vi "Retrieve Stored Session.vi"(8 "error in (no error)":errorcluster, 10 "Session in":refnum<class "Session.lvclass">, 11 "Client ID":string) -> (0 "error out":errorcluster, 1 "found":bool, 2 "Retrieved Session":refnum<class "Session.lvclass">)   [LabVIEW 2013, in "MQTT Server.lvlib" / "StoredSessions.lvclass"]
uses:
  StoredSessions.lvclass
  <vilib>/LabVIEW Open Source Project/MQTT Connection/MQTT_Base/Session/Session.lvclass
  <vilib>/LabVIEW Open Source Project/MQTT Connection/MQTT_Base/Session/Session State -- cluster.ctl
  <vilib>/LabVIEW Open Source Project/MQTT Control Packets/Control Packets/SUBSCRIBE/Topic Subscription -- cluster.ctl
  <vilib>/LabVIEW Open Source Project/MQTT Control Packets/Control Packets/ControlPacket/QualityOfService -- enum.ctl
  <vilib>/LabVIEW Open Source Project/MQTT Control Packets/Control Packets/ControlPacket/Pending Transmission -- cluster.ctl
  <vilib>/LabVIEW Open Source Project/MQTT Control Packets/Control Packets/ControlPacket/ControlPacket.lvclass
  <vilib>/LabVIEW Open Source Project/MQTT Connection/MQTT_Base/Session/Pending ACKs -- cluster.ctl
  <vilib>/LabVIEW Open Source Project/MQTT Connection/MQTT_Base/Session/Session.lvclass/Session.ctl
  <vilib>/LabVIEW Open Source Project/MQTT Control Packets/Control Packets/SUBSCRIBE/SUBSCRIBE.lvclass
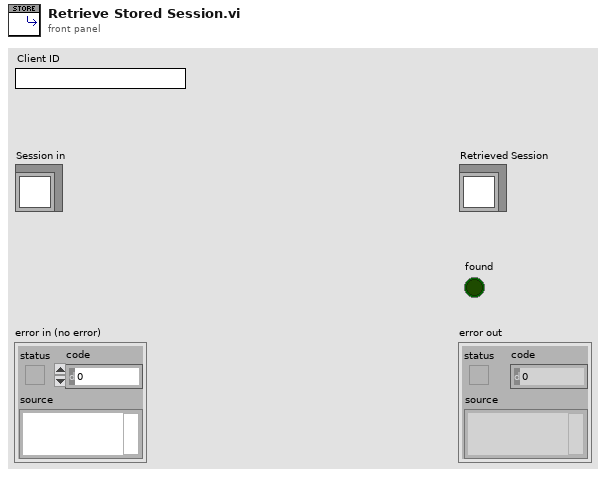
[diagram p1: front panel]
types:
  T1 = typedef "MQTT Base.lvlib/Session.lvclass/Session State -- cluster.ctl" = cluster{"CleanSession":bool, "Client ID":string, "Subscriptions":T2[], "Pending Transmissions":T4[], "Pending ACKs":T5[]}
  T2 = typedef "MQTT_Control_Packets.lvlib/SUBSCRIBE.lvclass/Topic Subscription -- cluster.ctl" = cluster{"Topic Filter":string, "QoS":T3}
  T3 = typedef "MQTT_Control_Packets.lvlib/ControlPacket.lvclass/QualityOfService -- enum.ctl" = enum16{"0 (At Most Once)", "1 (At Least Once)", "2 (Exactly Once)"}
  T4 = typedef "MQTT_Control_Packets.lvlib/ControlPacket.lvclass/Pending Transmission -- cluster.ctl" = cluster{"Message":refnum<class "ControlPacket.lvclass">, "QoS":T3, "Tx-Rx":bool}
  T5 = typedef "MQTT Base.lvlib/Session.lvclass/Pending ACKs -- cluster.ctl" = cluster{"Message":refnum<class "ControlPacket.lvclass">, "[ACK]":refnum<notifier>[], "Packet Identifier":u16}
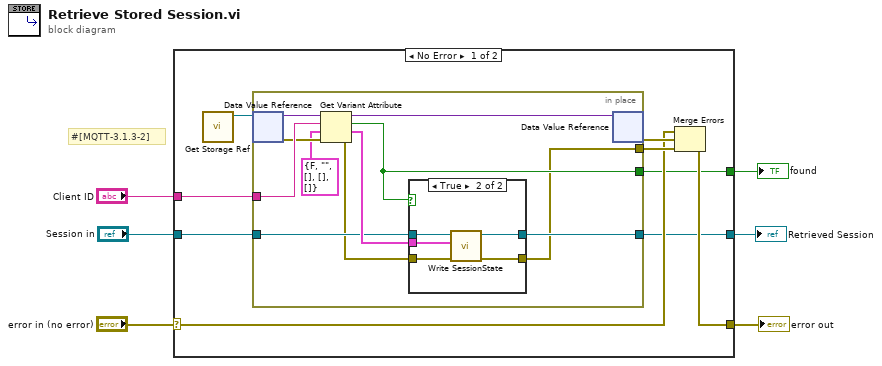
[diagram p0: block diagram]
diagram:
  # "#[MQTT-3.1.3-2]"
  n1 = case shown="No Error" "error in (no error)" {
    selector: "error in (no error)" -> [w11 w35]
    tunnel: [w10 w35] -> w5
    tunnel: "Client ID" -> [w14 _]
    tunnel: "Session in" -> [w9 w34]
    tunnel: [w8 _] -> w2
    tunnel: [w7 w34] -> w1
    frame No Error {
      n2 = call "Get Storage Ref.vi"() -> ("Storage"=w15:refnum<data-value>)  [unwired: 11 in]
      n3 = in-place {
        in-place-border: w14 -> [w25]
        in-place-border: [w16] -> w13
        in-place-border: w9 -> [w19]
        in-place-border: [w22] -> w8
        in-place-border: [w20] -> w7
        n4 = in-place-dvr #1(w15) -> (w26:variant, w23:errorcluster)
        n5 = Get Variant Attribute(Variant=w26, name=w25, default value (empty Variant)=T1 {"CleanSession"=FALSE, "Client ID"="", "Subscriptions"=[], "Pending Transmissions"=[], "Pending ACKs"=[]} ("Session State"), error in=w23) -> (duplicate Variant=w24:variant, found=w22:bool, value=w21:T1, error out=w17:errorcluster)
        n6 = case shown="True" w22 {
          tunnel: w21 -> [_ w32]
          tunnel: [w28 w31] -> w20
          tunnel: w19 -> [w28 w33]
          tunnel: w17 -> [w27 w30]
          tunnel: [w27 w29] -> w16
          frame False {
          }
          frame True {
            n7 = call <vilib>:"Write SessionState.vi"("error in (no error)"=w30, "Session State"=w32, "Session in"=w33) -> ("error out"=w29:errorcluster, "Session out"=w31:refnum<class "Session.lvclass">)  [unwired: 7 in]
          }
        }
        n8 = in-place-dvr #1(w24) -> (w12:errorcluster)  [unwired: 1 out]
      }
      n9 = Merge Errors(w11, w12, w13) -> (w10:errorcluster)
    }
    frame Error {
    }
  }
  "error out" <- w5
  "Retrieved Session" <- w1
  "found" <- w2
